vi "FPGAPowerMeasurement4withoutTrigger2.vi"() -> ()   [LabVIEW 2009]
uses:
  <vilib>/express/express analysis/Spectral/XNode/ExpressSpectralMeasurementsBlockNode.xnode
  <vilib>/express/express analysis/Spectral/Block/exnSpectralBlock spectral measurements peak poly.vi
  <vilib>/express/express analysis/Spectral/Block/exnSpectralBlock spectral measurements peak DDT.vi
panel:
  out "Waveform Graph 2":dynamicdata(graph)
  out "Waveform Graph":dynamicdata(graph)
  out "Average Voltage":dbl
  out "Voltage At Power":dynamicdata(graph)
  out "Voltage at FPGA":dynamicdata(graph)
  out "Power":dynamicdata(graph)
  out "Average Power":dbl
  out "Average Voltage":dbl
  out "Average Current":dbl
  out "Current":dynamicdata(graph)
  in  "stop":bool
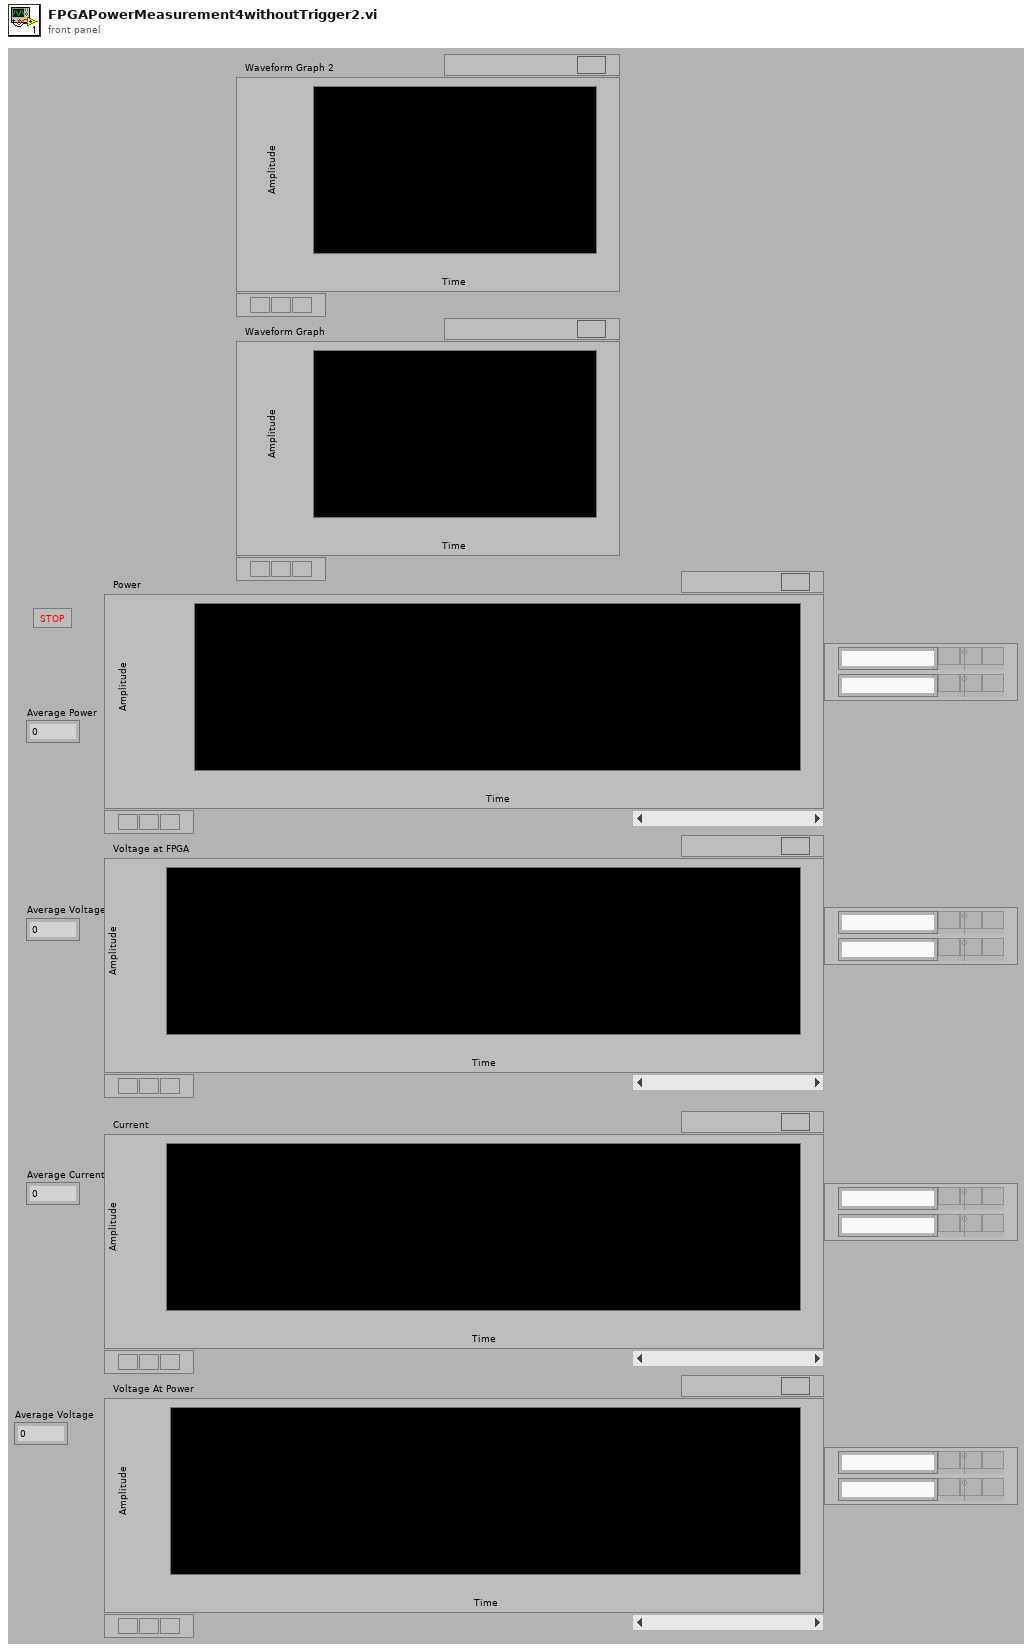
[diagram p1: front panel]
types:
  T1 = typedef "LVTextColorsTypeDef.ctl" = cluster{"Text Color":u32, "Background Color":u32}
  T2 = typedef "LVRangeTypeDef.ctl" = cluster{"Minimum":dbl, "Maximum":dbl, "Increment":dbl, "Minor Increment":dbl, "Start":dbl}
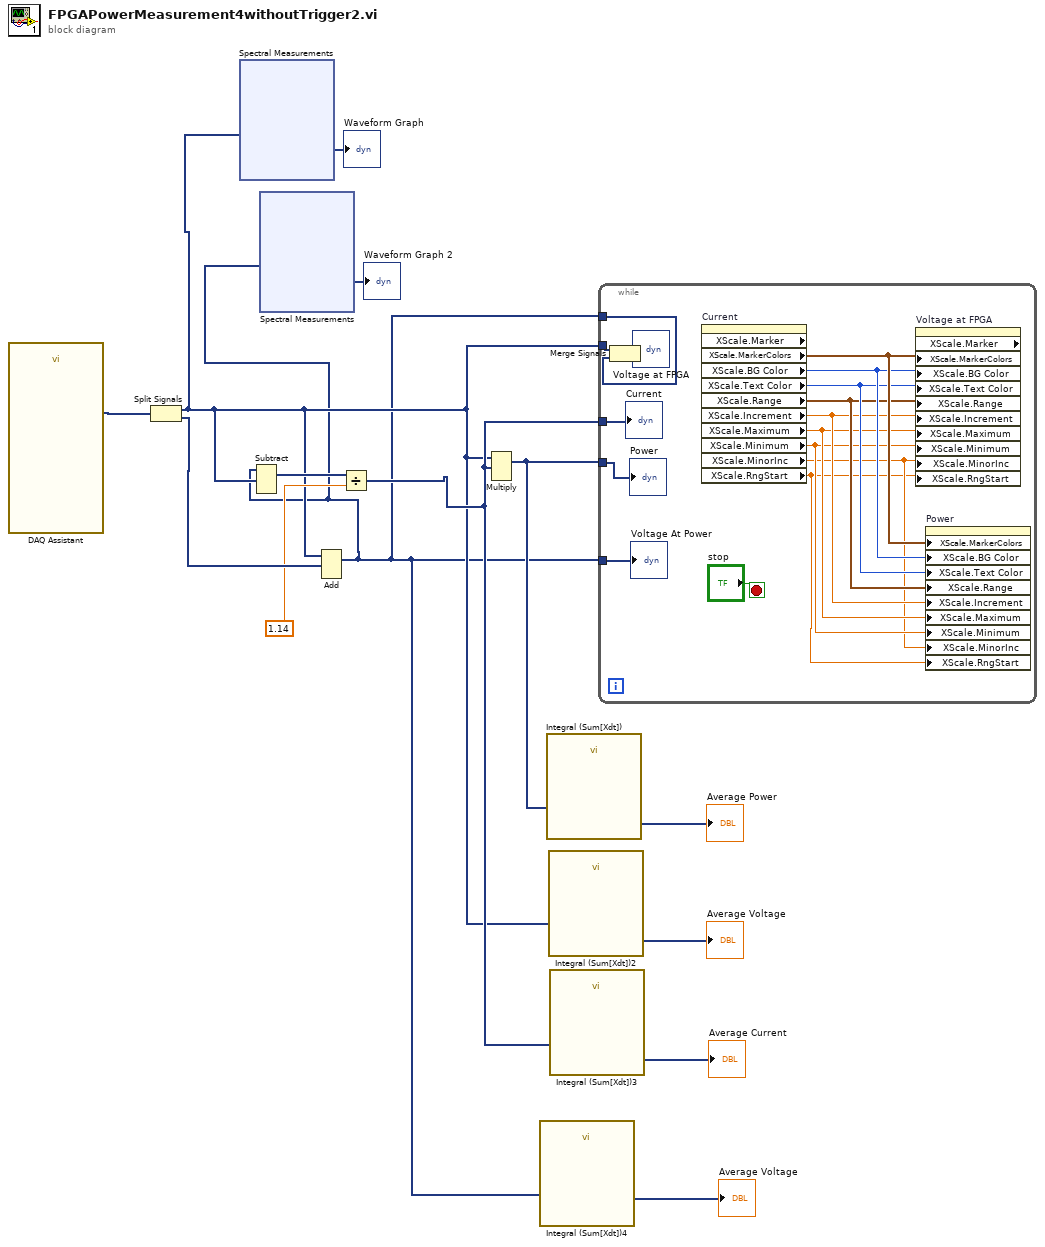
[diagram p0: block diagram]
diagram:
  n1 = call "DAQ Assistant"() -> ("data"=w10:dynamicdata)  [unwired: 17 in, 2 out]
  n2 = Split Signals(w10) -> (w2:dynamicdata, w9:dynamicdata)  [unwired: 2 in]
  n3 = xnode "Spectral Measurements"("Signals"=w2) -> ("FFT - (Peak)"=→"Waveform Graph":dynamicdata)  [unwired: 1 in, 2 out]
  n4 = Add(1:w9, 2:w2) -> (0:w1:dynamicdata)  [unwired: 1 in, 1 out]
  n5 = Subtract(1:w2, 2:w1) -> (0:w7:dynamicdata)  [unwired: 1 in, 1 out]
  n6 = xnode "Spectral Measurements"("Signals"=w1) -> ("FFT - (Peak)"=→"Waveform Graph 2":dynamicdata)  [unwired: 1 in, 2 out]
  n7 = Divide(x=w7, y=1.14) -> (x/y=w5:dynamicdata)
  n8 = Multiply(1:w5, 2:w2) -> (0:w14:dynamicdata)  [unwired: 1 in, 1 out]
  n9 = call "Integral (Sum[Xdt])4"("Signals"=w1) -> ("Result"=→"Average Voltage":dynamicdata)  [unwired: 5 in, 1 out]
  n10 = call "Integral (Sum[Xdt])"("Signals"=w14) -> ("Result"=→"Average Power":dynamicdata)  [unwired: 5 in, 1 out]
  n11 = call "Integral (Sum[Xdt])2"("Signals"=w2) -> ("Result"=→"Average Voltage":dynamicdata)  [unwired: 5 in, 1 out]
  n12 = call "Integral (Sum[Xdt])3"("Signals"=w5) -> ("Result"=→"Average Current":dynamicdata)  [unwired: 5 in, 1 out]
  n13 = while {
    tunnel: w2 -> [w28]
    tunnel: w5 -> [w29]
    tunnel: w14 -> [w27]
    tunnel: w1 -> [w17]
    tunnel: w1 -> [w15]
    stop <- "stop" stop-if-true
    n14 = Merge Signals(w28, w15) -> (→"Voltage at FPGA":dynamicdata)
    n15 = property on="Current" class="WFGraph (strict)" props=["XScale", "Marker", "XScale", "MarkerColors", "XScale", "BG Color", "XScale", "Text Color", "XScale", "Range", "XScale", "Increment", "XScale", "Maximum", "XScale", "Minimum", "XScale", "MinorInc", "XScale", "RngStart"]() -> ("XScale.MarkerColors"=w26:T1, "XScale.BG Color"=w25:u32, "XScale.Text Color"=w24:u32, "XScale.Range"=w23:T2, "XScale.Increment"=w22:dbl, "XScale.Maximum"=w21:dbl, "XScale.Minimum"=w20:dbl, "XScale.MinorInc"=w19:dbl, "XScale.RngStart"=w18:dbl)  [unwired: 2 in, 3 out]
    n16 = property on="Voltage at FPGA" class="WFGraph (strict)" props=["XScale", "Marker", "XScale", "MarkerColors", "XScale", "BG Color", "XScale", "Text Color", "XScale", "Range", "XScale", "Increment", "XScale", "Maximum", "XScale", "Minimum", "XScale", "MinorInc", "XScale", "RngStart"]("XScale.MarkerColors"=w26, "XScale.BG Color"=w25, "XScale.Text Color"=w24, "XScale.Range"=w23, "XScale.Increment"=w22, "XScale.Maximum"=w21, "XScale.Minimum"=w20, "XScale.MinorInc"=w19, "XScale.RngStart"=w18) -> ()  [unwired: 2 in, 3 out]
    n17 = property on="Power" class="WFGraph (strict)"("XScale.MarkerColors"=w26, "XScale.BG Color"=w25, "XScale.Text Color"=w24, "XScale.Range"=w23, "XScale.Increment"=w22, "XScale.Maximum"=w21, "XScale.Minimum"=w20, "XScale.MinorInc"=w19, "XScale.RngStart"=w18) -> ()  [unwired: 2 in, 2 out]
    "Current" <- w29
    "Power" <- w27
    "Voltage At Power" <- w17
  }
